vi "Get CD Item Property Value.vi"(8 "error in (no error)":errorcluster, 10 "CD Item Ref in":T1 format="%.0x", 11 "String Parameter in":refnum<class "String Parameter.lvclass">) -> (0 "error out":errorcluster, 3 "String Parameter out":refnum<class "String Parameter.lvclass">)   [LabVIEW 2019, in "CD Parameter Manager API.lvlib" / "String Parameter.lvclass"]
uses:
  String Parameter.lvclass
  C:/Repositories/CSD_Custom_Device/CSD_Custom_Device/Source/Libraries/CD Parameter Manager API/Parameter Class/Parameter.lvclass
  <vilib>/NI VeriStand/Custom Device API/Custom Device Item Ref.ctl
  Parameter Class/Parameter.lvclass/Parameter.ctl
  String Parameter.lvclass/String Parameter.ctl
  Parameter Class/Member Accessors/Read Control label.vi
  Member Accessors/Read Value.vi
  Member Accessors/Write Value.vi
  <vilib>/NI VeriStand/Custom Device API/Get Item Property (String).vi
  <vilib>/NI VeriStand/Custom Device API/Custom Device API.lvlib
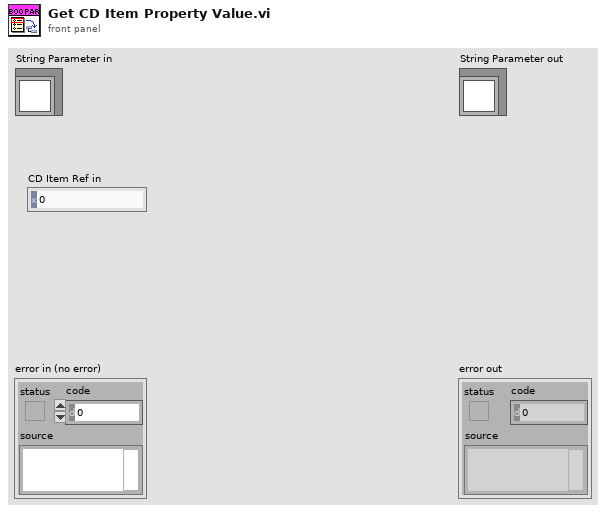
[diagram p1: front panel]
types:
  T1 = typedef "Custom Device API.lvlib/Custom Device Item Ref.ctl" = u64
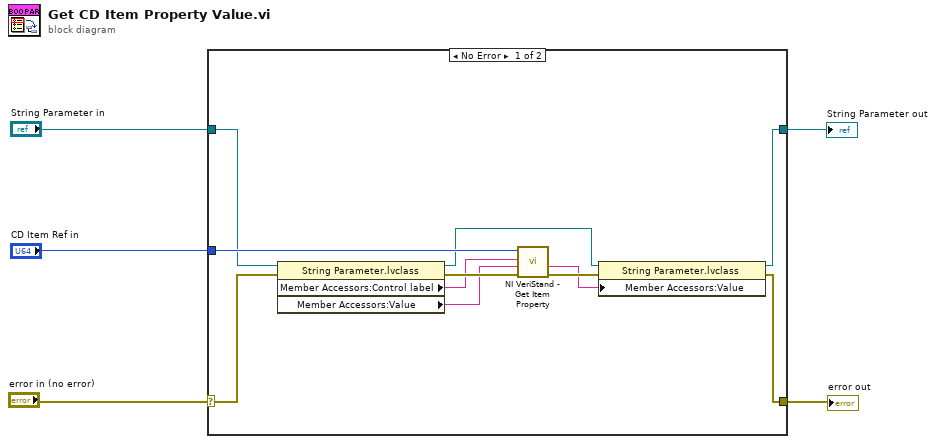
[diagram p0: block diagram]
diagram:
  n1 = case shown="No Error" "error in (no error)" {
    selector: "error in (no error)" -> [w15 w17]
    tunnel: [w10 w17] -> w4
    tunnel: "CD Item Ref in" -> [w16 _]
    tunnel: [w6 w18] -> w3
    tunnel: "String Parameter in" -> [w7 w18]
    frame No Error {
      n2 = property class="String Parameter.lvclass"(reference=w7, error in=w15) -> (reference out=w8:refnum<class "String Parameter.lvclass">, error out=w14:errorcluster, "Member Accessors:Control label"=w13:string, "Member Accessors:Value"=w12:string)
      n3 = call-poly <vilib>:"NI VeriStand - Get Item Property.vi"("error in (no error)"=w14, "Default Value"=w12, "Property Name"=w13, "Item Ref in"=w16) -> ("error out"=w11:errorcluster, "Value"=w9:string)  [unwired: 4 in, 2 out]
      n4 = property class="String Parameter.lvclass"(reference=w8, error in=w11, "Member Accessors:Value"=w9) -> (reference out=w6:refnum<class "String Parameter.lvclass">, error out=w10:errorcluster)
    }
    frame Error {
    }
  }
  "error out" <- w4
  "String Parameter out" <- w3
